vi "SV Multitone THD IMD SNR (Time) (1 Ch).vi"(0 "response signal [EU]":waveform(dbl), 1 "reference tones":T4(array[cluster]) {"phase (deg)" format="%0.3p"; "amplitude [EU pk]" format="%0.3p"; "frequency [Hz]" format="%0.3p"}, 2 "frequency range [Hz]":cluster{"start":dbl, "stop":dbl}={"start"=-1.0, "stop"=-1.0} {"stop" format="%.2f"; "start" format="%.2f"}, 3 "advanced span [Hz]":dbl=-1.0 format="%.2f", 5 "error in (no error)":errorcluster, 6 "desired units":T5={"THD"=enum."dB", "IMD"=enum."dB", "SNR"=enum."dB", "harmonic level"=enum."EU rms", "intermodulation level"=enum."EU rms", "noise level"=enum."EU rms"}, 7 "configuration":T3={"maximum harmonic"=5, "IMD proxy frequencies"=[], "noise proxy"=0} {"noise proxy" items=["Residual"=0, "L50"=50, "L75"=75, "L90"=90, "Odd bins"=13579]}) -> (12 "unit labels":T6, 13 "distortion frequencies [Hz]":T1, 14 "complex spectrum response":T13={"complex spectrum response"={"f0"=0.0, "df"=1.0, "complex spectrum"=[]}, "spectrum info"={"channel name"="", "description"="", "x-axis units"=0, "spectral info"={"spectrum type"=enum."Power [Magnitude^2]", "linear/dB"=enum."linear", "window"=0, "window size"=0, "FFT size"=0}, "engineering units"=0, "custom label"="", "dB reference [EU]"=0.0, "peak units"=enum."rms", "weighting filter"=0, "spectral density?"=FALSE, "unit label"="", "spectrum skewed?"=FALSE, "complimentary spectrum units"=enum."none"}} {"spectrum info"."x-axis units" items=["Time (s)"=0, "Frequency-CB (Hz)"=1, "Frequency-CPB (Hz)"=1248, "Frequency-Arbitrary (Hz)"=2357, "Quefrency (s)"=2, "Revolutions (rev)"=3, "Order"=4, "Speed (RPM)"=11, "Speed (rad/s)"=21, "Index"=65535]; "spectrum info"."weighting filter" items=["Linear", "A-weighting", "B-weighting", "C-weighting", "ITU-R 468-4", "Dolby", "CCITT", "C-message", "Wb", "Wc", "Wd", "We", "Wf", "Wh", "Wj", "Wk", "Wm", "AES17 20 kHz lowpass", "AES17 40 kHz lowpass", "AES17 20 kHz highpass", "AES17 40 kHz highpass"]; "spectrum info"."dB reference [EU]" format="%.2f"; "spectrum info"."engineering units" items=["custom..."=0, "V"=1, "A"=21, "C"=30, "pC"=31, "s"=32, "-"=29, "Pa"=2, "N"=20, "g"=3, "m/s^2"=4, "m/s"=5, "m"=6, "mm/s"=12, "mm"=13, "micron/s"=14, "micron"=15, "in/s^2"=7, "in/s"=8, "in"=9, "mil/s"=10, "mil"=11, "rad/s^2"=16, "rad/s"=17, "rad"=18, "deg/s^2"=26, "deg/s"=27, "deg"=28, "RPM"=22, "cycle/s^2"=23, "Hz"=24, "cycle"=25, "strain"=19]; "spectrum info"."spectral info"."window" items=["None "=0, "Hanning"=1, "Hamming"=2, "Blackman-Harris"=3, "Exact Blackman"=4, "Blackman"=5, "Flat Top"=6, "4 Term B-Harris "=7, "7 Term B-Harris"=8, "Low Sidelobe"=9, "Force - Exponential"=10, "Gaussian"=62]; "complex spectrum response"."complex spectrum" format="%.2f"; "complex spectrum response"."df" format="%.2f"; "complex spectrum response"."f0" format="%.2f"}, 15 "THD":dbl format="%.2f", 16 "IMD":dbl format="%.2f", 17 "SNR":dbl format="%.2f", 18 "levels":T14 {"noise" format="%.2f"; "intermodulation" format="%.2f"; "harmonic" format="%.2f"}, 19 "error out":errorcluster)   [LabVIEW 2017, in "SoundVib_Multitone.lvlib"]
doc: "Performs total harmonic distortion (THD), intermodulation distortion (IMD), and signal-to-noise ratio (SNR) measurements, including measuring the fundamental tones, harmonic components, intermodulation components, and residual noise. Wire data to the <B>scaled signal [EU]</B> input to determine the polymorphic instance to use or manually select the instance."
uses:
  <vilib>/addons/Sound and Vibration/svt_Multitone Distortion/SoundVib_Multitone.lvlib
  <vilib>/addons/_NISVFA/_Shared subVIs/Controls/svc_Spectrum Info.ctl
  <vilib>/addons/_NISVFA/_Shared subVIs/Controls/svc_X-Axis Units.ctl
  <vilib>/addons/_NISVFA/_Shared subVIs/Controls/svc_Spectrum Type.ctl
  <vilib>/addons/_NISVFA/_Shared subVIs/Controls/svc_Engineering Units Text Ring.ctl
  <vilib>/addons/_NISVFA/_Shared subVIs/Controls/svc_Weighting Filter Text Ring.ctl
  <vilib>/addons/_NISVFA/_Shared subVIs/Controls/svc_Complimentary Spectrum Units.ctl
  <vilib>/addons/_NISVFA/_Shared subVIs/Controls/svc_Noise Proxy.ctl
  <vilib>/addons/_NISVFA/_Shared subVIs/Controls/svc_Window.ctl
  <vilib>/addons/Sound and Vibration/svt_Distortion/SoundVib_Distortion.lvlib
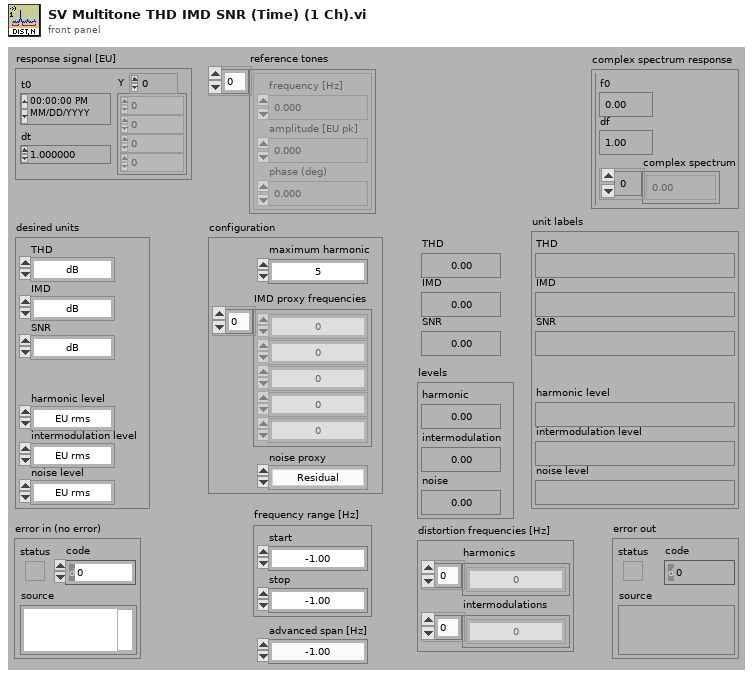
[diagram p1: front panel]
types:
  T1 = cluster{"harmonics":dbl[], "intermodulations":dbl[]}
  T2 = typedef "svc_Noise Proxy.ctl" = u16
  T3 = cluster{"maximum harmonic":i32, "IMD proxy frequencies":dbl[], "noise proxy":T2}
  T4 = cluster{"frequency [Hz]":dbl, "amplitude [EU pk]":dbl, "phase (deg)":dbl}[]
  T5 = cluster{"THD":enum16{"dB", "linear ratio", "%"}, "IMD":enum16{"dB", "linear ratio", "%"}, "SNR":enum16{"dB", "linear ratio", "%"}, "harmonic level":enum16{"EU^2 rms", "EU rms", "dB", "dBc", "dBV", "dBu", "dBm"}, "intermodulation level":enum16{"EU^2 rms", "EU rms", "dB", "dBc", "dBV", "dBu", "dBm"}, "noise level":enum16{"EU^2 rms", "EU rms", "dB", "dBc", "dBV", "dBu", "dBm"}}
  T6 = cluster{"THD":string, "IMD":string, "SNR":string, "harmonic level":string, "intermodulation level":string, "noise level":string}
  T7 = typedef "svc_Spectrum Info.ctl" = cluster{"channel name":string, "description":string, "x-axis units":T8, "spectral info":cluster{"spectrum type":T9, "linear/dB":enum16{"linear", "dB"}, "window":u16, "window size":i32, "FFT size":i32}, "engineering units":T10, "custom label":string, "dB reference [EU]":dbl, "peak units":enum16{"rms", "peak", "peak-peak"}, "weighting filter":T11, "spectral density?":bool, "unit label":string, "spectrum skewed?":bool, "complimentary spectrum units":T12}
  T8 = typedef "svc_X-Axis Units.ctl" = u16
  T9 = typedef "svc_Spectrum Type.ctl" = enum16{"FFT Spectrum [complex]", "Amplitude [Magnitude]", "Power [Magnitude^2]", "Cross Spectrum [complex]", "Frequency Response [Complex]"}
  T10 = typedef "svc_Engineering Units Text Ring.ctl" = u16
  T11 = typedef "svc_Weighting Filter Text Ring.ctl" = u16
  T12 = typedef "svc_Complimentary Spectrum Units.ctl" = enum16{"none", "radians", "degrees", "cycles", "imaginary"}
  T13 = cluster{"complex spectrum response":cluster{"f0":dbl, "df":dbl, "complex spectrum":cdb[]}, "spectrum info":T7}
  T14 = cluster{"harmonic":dbl, "intermodulation":dbl, "noise":dbl}
  T15 = typedef "svc_Window.ctl" = u32
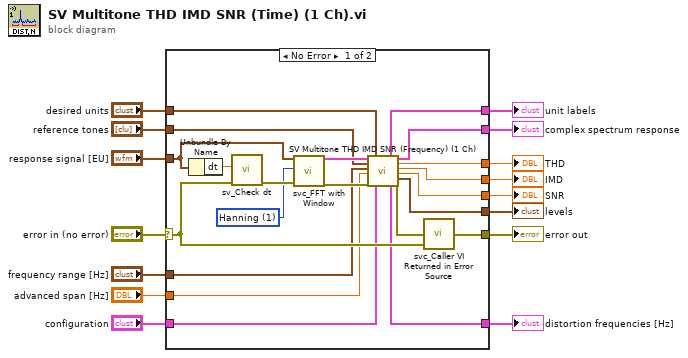
[diagram p0: block diagram]
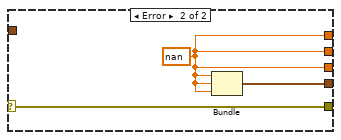
[diagram p2: hidden frame]
diagram:
  n1 = case shown="No Error" "error in (no error)" {
    selector: "error in (no error)" -> [w25 w39]
    tunnel: "response signal [EU]" -> [w27 _]
    tunnel: [w30 w39] -> w14
    tunnel: [w24 w38] -> w1
    tunnel: [w34 _] -> w12
    tunnel: [w33 _] -> w11
    tunnel: "desired units" -> [w32 _]
    tunnel: "reference tones" -> [w23 _]
    tunnel: "frequency range [Hz]" -> [w22 _]
    tunnel: "configuration" -> [w17 _]
    tunnel: [w21 w37] -> w6
    tunnel: [w20 w37] -> w5
    tunnel: [w19 w37] -> w4
    tunnel: [w18 _] -> w3
    tunnel: "advanced span [Hz]" -> [w16 _]
    frame No Error {
      w28 = T15 1 items=["None ", "Hanning", "Hamming", "Blackman-Harris", "Exact Blackman", "Blackman", "Flat Top", "4 Term B-Harris ", "7 Term B-Harris", "Low Sidelobe", "Force - Exponential", "Gaussian"] ("window")
      n2 = Unbundle By Name(w27) -> ("dt"=w26:dbl)
      n3 = call <vilib>:"sv_Check dt.vi"("error in"=w25, "dt"=w26) -> ("error out"=w29:errorcluster)  [unwired: 8 in, 1 out]
      n4 = call <vilib>:"svc_FFT with Window.vi"("time signal in [EU]"=w27, "window"=w28, "error in (no error)"=w29) -> ("complex spectrum"=w36:T13, "error out"=w35:errorcluster)  [unwired: 15 in]
      n5 = call <vilib>:"SV Multitone THD IMD SNR (Frequency) (1 Ch).vi"("complex spectrum response"=w36, "reference tones"=w23, "frequency range [Hz]"=w22, "advanced span [Hz]"=w16, "error in (no error)"=w35, "desired units"=w32, "configuration"=w17) -> ("unit labels"=w34:T6, "distortion frequencies [Hz]"=w18:T1, "complex spectrum response"=w33:T13, "THD"=w21:dbl, "IMD"=w20:dbl, "SNR"=w19:dbl, "levels"=w24:T14, "error out"=w31:errorcluster)  [unwired: 5 in]
      n6 = call <vilib>:"svc_Caller VI Returned in Error Source.vi"("warning input to caller"=w25, "error in (no error)"=w31) -> ("error out"=w30:errorcluster)  [unwired: 3 in]
    }
    frame Error {
      w37 = nan ("SINAD")
      n7 = Bundle("SINAD"=w37, "SINAD"=w37, "SINAD"=w37) -> (w38:cluster{"SINAD":dbl, "SINAD":dbl, "SINAD":dbl})  [unwired: 1 in]
    }
  }
  "error out" <- w14
  "levels" <- w1
  "complex spectrum response" <- w11
  "unit labels" <- w12
  "distortion frequencies [Hz]" <- w3
  "THD" <- w6
  "IMD" <- w5
  "SNR" <- w4
